vi "Insert Chan Grp.vi"(7 "Insert to Prev Place? (T)":bool=TRUE, 8 "error in (no error)":errorcluster, 9 "ChanGroupPos":i32, 10 "ChanGrp to Add":refnum<class "ChanGrp.lvclass">, 11 "TimingGrp in":refnum<class "TimingGrp.lvclass">) -> (0 "error out":errorcluster, 1 "ChanGroupPos":i32, 3 "TimingGrp out":refnum<class "TimingGrp.lvclass">)   [LabVIEW 2012, in "Configuration Grandmaster.lvlib" / "TimingGrp.lvclass"]
uses:
  TimingGrp.lvclass
  Class Chan Group/ChanGrp.lvclass
  TimingGrp.lvclass/TimingGrp.ctl
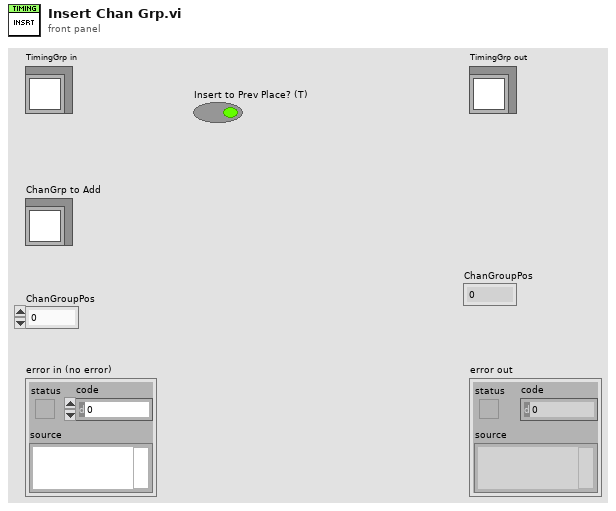
[diagram p1: front panel]
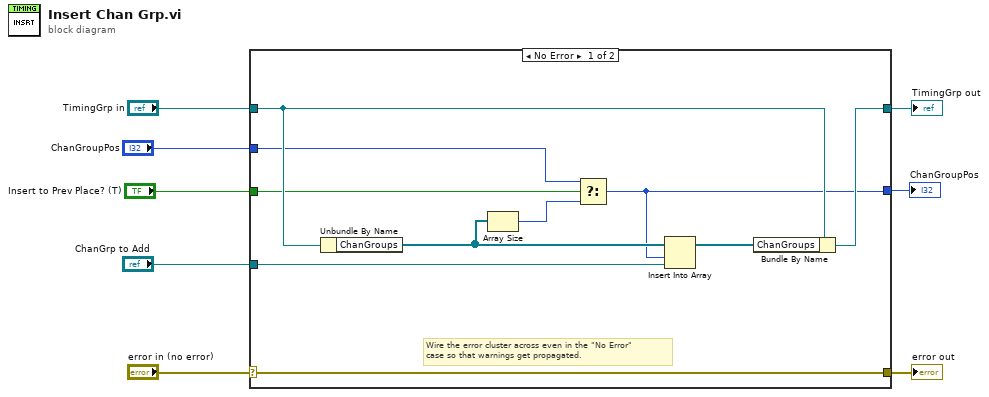
[diagram p0: block diagram]
diagram:
  n1 = case shown="No Error" "error in (no error)" {
    selector: "error in (no error)" -> [w18 w21]
    tunnel: [w18 w21] -> w7
    tunnel: [w13 w20] -> w5
    tunnel: "TimingGrp in" -> [w15 w20]
    tunnel: "ChanGrp to Add" -> [w17 _]
    tunnel: "ChanGroupPos" -> [w11 w19]
    tunnel: "Insert to Prev Place? (T)" -> [w12 _]
    tunnel: [w10 w19] -> w1
    frame No Error {
      # "Wire the error cluster across even in the \"No Error\"\ncase so that warnings get propagated."
      n2 = Unbundle By Name(w15) -> ("ChanGroups"=w16:refnum<class "ChanGrp.lvclass">[])
      n3 = Array Size(array=w16) -> (size(s)=w9:i32)
      n4 = Select(t=w11, s=w12, f=w9) -> (s? t:f=w10:i32)
      n5 = Insert Into Array(array=w16, index=w10, new element=w17) -> (w14:refnum<class "ChanGrp.lvclass">[])
      n6 = Bundle By Name(cluster=w15, "ChanGroups"=w14) -> (w13:refnum<class "TimingGrp.lvclass">)
    }
    frame Error {
    }
  }
  "error out" <- w7
  "TimingGrp out" <- w5
  "ChanGroupPos" <- w1
